vi "zeroMQ-publish-ADR-50mK.vi"() -> ()   [LabVIEW 2016]
uses:
  <vilib>/addons/zeromq/socket_type.ctl
  <vilib>/addons/zeromq/zmq_context.lvclass
  <vilib>/addons/zeromq/zmq_socket.lvclass
  <vilib>/addons/zeromq/zeromq.lvlib
panel:
  out "ADR 50mK (sent message)":dbl format="%#_8g"
  in  "STOP !!":bool
  out "Publishing":bool
  # "Publishes the 50mK temperature from the StarCryo ADR control software (NI shared variable) every second to port 5555 via zeroMQ. Connect with client to get temp."
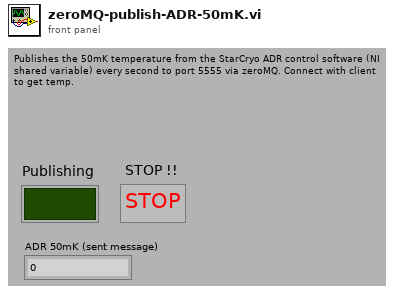
[diagram p1: front panel]
types:
  T1 = typedef "zeromq.lvlib/socket_type.ctl" = enum8{"ZMQ_PAIR", "ZMQ_PUB", "ZMQ_SUB", "ZMQ_REQ", "ZMQ_REP", "ZMQ_DEALER", "ZMQ_ROUTER", "ZMQ_PULL", "ZMQ_PUSH", "ZMQ_XPUB", "ZMQ_XSUB"}
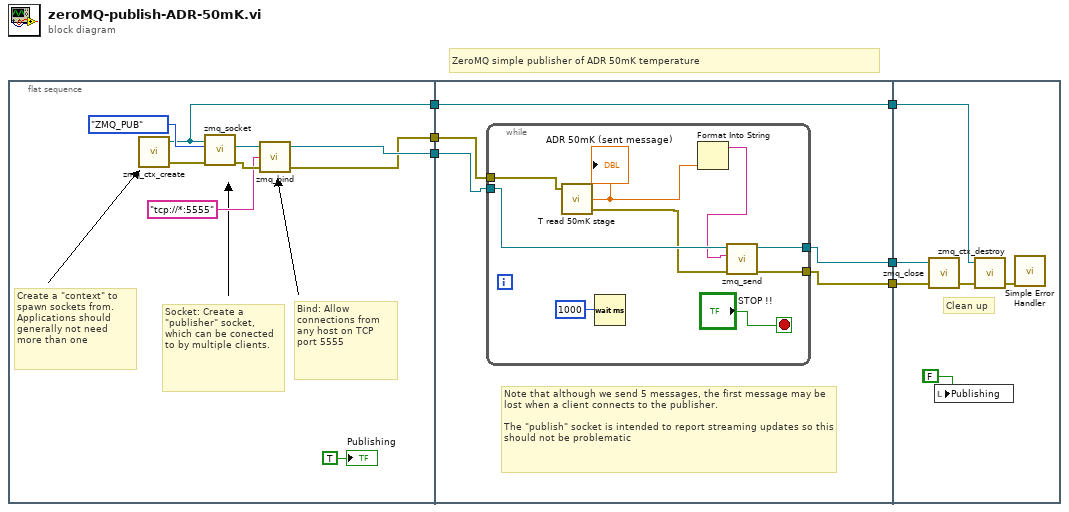
[diagram p0: block diagram]
diagram:
  # "ZeroMQ simple publisher of ADR 50mK temperature"
  n1 = flat-sequence {
    tunnel: [w10] -> w6
    tunnel: [w9] -> w5
    tunnel: [w8] -> w3
    tunnel: w6 -> [w19]
    tunnel: w5 -> [w18]
    tunnel: [w20] -> w4
    tunnel: w3 -> [w20]
    tunnel: [w17] -> w2
    tunnel: [w16] -> w1
    tunnel: w4 -> [w33]
    tunnel: w2 -> [w32]
    tunnel: w1 -> [w31]
    frame #0 {
      # "Bind: Allow connections from any host on TCP port 5555"
      # "Socket: Create a \"publisher\" socket, which can be conected to by multiple clients."
      # "Create a \"context\" to spawn sockets from. Applications should generally not need more than one"
      n2 = call <vilib>:"zmq_ctx_create.vi"() -> ("error out"=w14:errorcluster, "context out"=w8:refnum<class "zmq_context.lvclass">)  [unwired: 4 in]
      n3 = call <vilib>:"zmq_socket.vi"("error in"=w14, "socket type"=socket_type."ZMQ_PUB", "context in"=w8) -> ("error out"=w13:errorcluster, "socket out"=w11:refnum<class "zmq_socket.lvclass">)  [unwired: 2 in, 1 out]
      n4 = call <vilib>:"zmq_bind.vi"("error in"=w13, "endpoint"="tcp://*:5555", "socket in"=w11) -> ("error out"=w9:errorcluster, "socket out"=w10:refnum<class "zmq_socket.lvclass">)  [unwired: 1 in]
      "Publishing" <- TRUE ("Publishing")
    }
    frame #1 {
      # "Note that although we send 5 messages, the first message may be lost when a client connects to the publisher.\n\nThe \"publish\" socket is intended to report streaming updates so this should not be problematic"
      n5 = while {
        tunnel: [w29] -> w17
        tunnel: [w27] -> w16
        tunnel: w19 -> [w25]
        tunnel: w18 -> [w23]
        stop <- "STOP !!" stop-if-true
        n6 = call <userlib>:"T read 50mK stage.vi"("error in (no error)"=w23) -> ("error out"=w21:errorcluster, "ADR 50mK [K] (921)"=w22:dbl)
        "ADR 50mK (sent message)" <- w22
        n7 = Wait (ms)(milliseconds to wait=u32 1000) -> ()  [unwired: 1 out]
        n8 = Format Into String(w22) -> (resulting string=w24:string)  [unwired: 3 in, 1 out]
        n9 = call <vilib>:"zmq_send.vi"("error in"=w21, "data"=w24, "socket in"=w25) -> ("error out"=w27:errorcluster, "socket out"=w29:refnum<class "zmq_socket.lvclass">)  [unwired: 4 in]
      }
    }
    frame #2 {
      (unwired) FALSE ("Acquiring")
      # "Clean up"
      n10 = call <vilib>:"zmq_close.vi"("error in"=w31, "socket"=w32) -> ("error out"=w34:errorcluster)  [unwired: 3 in]
      n11 = local write "Publishing"(FALSE ("Acquiring")) -> ()
      n12 = call <vilib>:"zmq_ctx_destroy.vi"("error in"=w34, "context in"=w33) -> ("error out"=w35:errorcluster)  [unwired: 3 in]
      n13 = call <vilib>:"Simple Error Handler.vi"("error in (no error)"=w35) -> ()  [unwired: 4 in, 5 out]
    }
  }
